vi "Acquire Zero Correct.vi"(0 "VISA resource name":refnum<visa-resource-name>, 11 "error in (no error)":errorcluster) -> (4 "VISA resource name out":refnum<visa-resource-name>, 15 "error out":errorcluster)   [LabVIEW 2020, in "Keithley 648X Series.lvlib"]
doc: "Sets the value for the zero correction of the current current range. The value used is the internal offset measured upon usage. After execution zero check will be disabled and zero correct will be enabled.\n\n<b>Note:</b>\nConfigure the desired current range using the <b>Configure Range</b> VI. Also, the zero correct value will need to be reacquired if changing the current setting to a range lower than the current range configured at the time of the zero correct acquisition."
uses:
  <instrlib>/Keithley 648X Series/Keithley 648X Series.lvlib
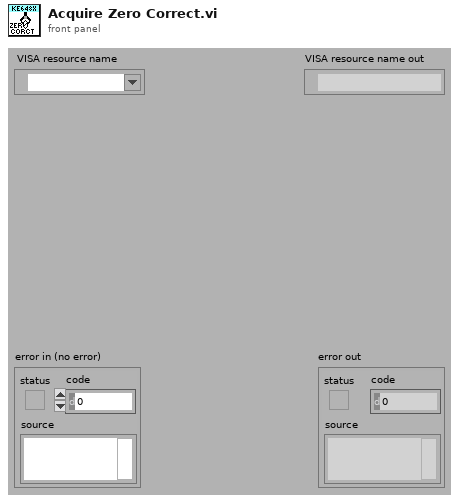
[diagram p1: front panel]
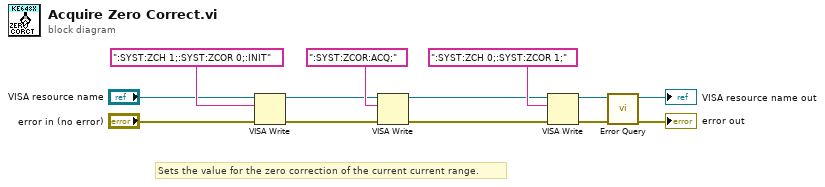
[diagram p0: block diagram]
diagram:
  # "Sets the value for the zero correction of the current current range."
  n1 = VISA Write(VISA resource name="VISA resource name", write buffer=":SYST:ZCH 1;:SYST:ZCOR 0;:INIT", error in (no error)="error in (no error)") -> (VISA resource name out=w10:refnum<visa-resource-name>, error out=w3:errorcluster)  [unwired: 1 out]
  n2 = VISA Write(VISA resource name=w10, write buffer=":SYST:ZCOR:ACQ;", error in (no error)=w3) -> (VISA resource name out=w7:refnum<visa-resource-name>, error out=w4:errorcluster)  [unwired: 1 out]
  n3 = VISA Write(VISA resource name=w7, write buffer=":SYST:ZCH 0;:SYST:ZCOR 1;", error in (no error)=w4) -> (VISA resource name out=w6:refnum<visa-resource-name>, error out=w5:errorcluster)  [unwired: 1 out]
  n4 = call <instrlib>:"Error Query.vi"("error in (no error)"=w5, "VISA resource name"=w6) -> ("error out"=→"error out":errorcluster, "VISA resource name out"=→"VISA resource name out":refnum<visa-resource-name>)  [unwired: 6 in, 2 out]
